vi "Send Software Advanced Trigger [AT].vi"(8 "error in (no error)":errorcluster, 11 "CS++Fgen in":refnum<class "CS++Fgen.lvclass">) -> (0 "error out":errorcluster, 3 "CS++Fgen out":refnum<class "CS++Fgen.lvclass">)   [LabVIEW 2013, in "CS++Fgen.lvlib" / "CS++Fgen.lvclass"]
doc: "This VI sends a software-generated advance trigger to the function generator. If the trigger source is not set to software trigger, this VI returns the error IVIFGEN_ERROR_TRIGGER_NOT_SOFTWARE.\n\nNotes:\n\n(1) This VI does not normally check the instrument status. Typically, you call this VI only in a sequence of calls to other low-level driver VIs. The sequence performs one operation. You use the low-level VIs to optimize one or more aspects of interaction with the instrument. If you want to check the instrument status, call the IviFgen Error-Query VI at the conclusion of the sequence.\n\n(2) This VI is part of the IviFgenAdvanceTrigger [AT] extension group."
uses:
  CS++Fgen.lvclass
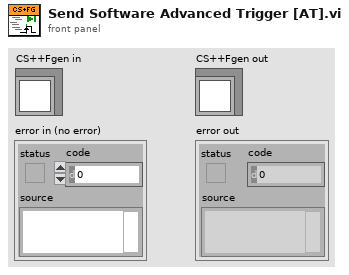
[diagram p1: front panel]
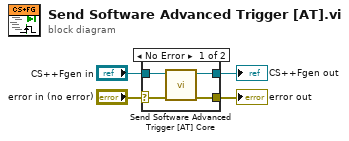
[diagram p0: block diagram]
diagram:
  n1 = case shown="No Error" "error in (no error)" {
    selector: "error in (no error)" -> [w6 w10]
    tunnel: [w5 w10] -> w3
    tunnel: [w7 w9] -> w1
    tunnel: "CS++Fgen in" -> [w8 w9]
    frame No Error {
      n2 = call-dynamic "Send Software Advanced Trigger [AT] Core.vi"("error in (no error)"=w6, "CS++Fgen in"=w8) -> ("error out"=w5:errorcluster, "CS++Fgen out"=w7:refnum<class "CS++Fgen.lvclass">)  [unwired: 8 in]
    }
    frame Error {
    }
  }
  "error out" <- w3
  "CS++Fgen out" <- w1
